vi "ALTS-2015 Read Last User.vi"(6 "Read?":bool, 8 "error in (no error)":errorcluster, 11 "Last User":string) -> (0 "error out":errorcluster, 3 "Last User":string)   [LabVIEW 2013]
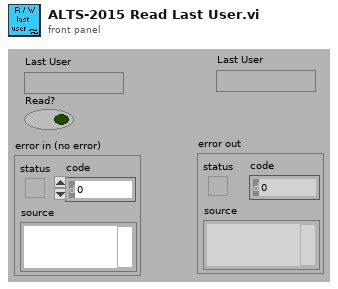
[diagram p1: front panel]
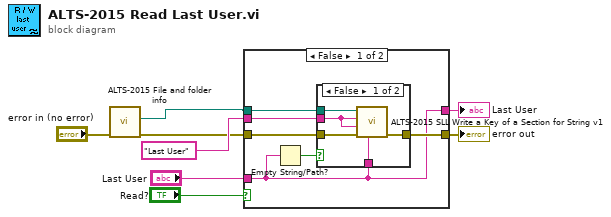
[diagram p0: block diagram]
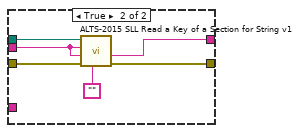
[diagram p3: hidden frame]
diagram:
  n1 = call "ALTS-2015 File and folder info.vi"("error in (no error)"="error in (no error)") -> ("error out"=w2:errorcluster, "INI file path"=w1:path)  [unwired: 5 in, 4 out]
  n2 = case shown="False" "Read?" {
    tunnel: w1 -> [w14 w26]
    tunnel: w2 -> [w12 w25]
    tunnel: "Last User" ("Section") -> [w13 w24]
    tunnel: [w11 w22] -> w6
    tunnel: "Last User" -> [w9 _]
    tunnel: [w9 w21] -> w4
    frame False {
      n3 = Empty String/Path?(string/path=w9) -> (empty?=w10:bool)
      n4 = case shown="False" w10 {
        tunnel: w14 -> [w19 _]
        tunnel: w13 -> [w18 _]
        tunnel: w12 -> [w17 w20]
        tunnel: [w16 w20] -> w11
        tunnel: w9 -> [w15 _]
        frame False {
          n5 = call "ALTS-2015 SLL Write a Key of a Section for String v1.vi"("Key Value"=w15, "error in (no error)"=w17, "Key Name"=w18, "Section"=w18, "Application INI file path"=w19) -> ("error out"=w16:errorcluster)  [unwired: 6 in]
        }
        frame True {
        }
      }
    }
    frame True {
      n6 = call "ALTS-2015 SLL Read a Key of a Section for String v1.vi"("Key Data Type"="", "error in (no error)"=w25, "Key Name"=w24, "Section"=w24, "INI File Path"=w26) -> ("error out"=w22:errorcluster, "Key Value"=w21:string)  [unwired: 5 in]
    }
  }
  "error out" <- w6
  "Last User" <- w4
